vi "Query Outputs.vi"(8 "error in":errorcluster, 11 "PIOD in":refnum<class "PIOD.lvclass">) -> (0 "error out":errorcluster, 3 "PIOD out":refnum<class "PIOD.lvclass">)   [LabVIEW 2018, in "PIOD.lvlib" / "PIOD.lvclass"]
uses:
  PIOD.lvclass
  Custom Controls/File Number.ctl
  PIOD.lvclass/PIOD.ctl
  Accessors/Read/Read Timeout (ms).vi
  <vilib>/ethernetip/ethernetip.llb/EthernetIP SLC500 Read Bit.vi
  <vilib>/ethernetip/ethernetip.lvlib
  PPLs/PLC/Parent/PLC.lvlibp/PLC.lvclass
  C:/AME Test Engineering/LabVIEW/PPLs/PLC/Parent/PLC.lvlibp/PLC.lvclass
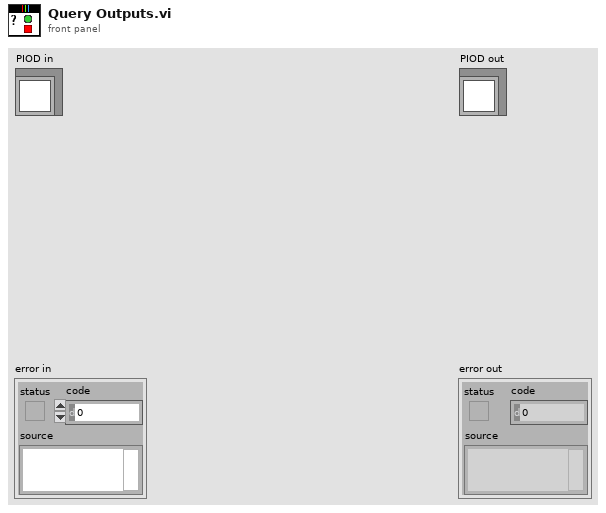
[diagram p1: front panel]
types:
  T1 = typedef "PIOD.lvlib/PIOD.lvclass/File Number.ctl" = enum16{"Output", "Input", "Status", "Output2"}
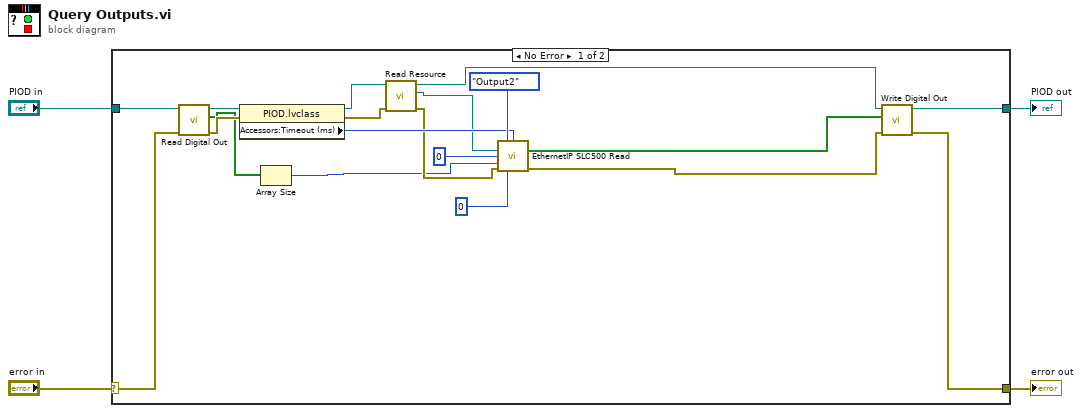
[diagram p0: block diagram]
diagram:
  n1 = case shown="No Error" "error in" {
    selector: "error in" -> [w11 w25]
    tunnel: [w20 w25] -> w3
    tunnel: [w21 w24] -> w1
    tunnel: "PIOD in" -> [w12 w24]
    frame No Error {
      n2 = call "Read Digital Out.vi"("error in"=w11, "PLC in"=w12) -> ("error out"=w9:errorcluster, "Digital Out"=w8:bool[], "PLC out"=w10:refnum<class "PIOD.lvclass">)  [unwired: 7 in]
      n3 = property class="PIOD.lvclass"(reference=w10, error in=w9) -> (reference out=w18:refnum<class "PIOD.lvclass">, error out=w19:errorcluster, "Accessors:Timeout (ms)"=w22:i32)
      n4 = Array Size(array=w8) -> (size(s)=w6:i32)
      n5 = call "Read Resource.vi"("error in (no error)"=w19, "PLC in"=w18) -> ("error out"=w15:errorcluster, "Resource"=w16:refnum<visa-resource-name>, "PLC out"=w17:refnum<class "PIOD.lvclass">)  [unwired: 7 in]
      n6 = call-poly <vilib>:"EthernetIP SLC500 Read.vi"("File Number"=File_Number."Output2", "Timeout (ms)"=w22, "Network Path"=w16, "Element Number"=u16 0, "Number of Bits"=w6, "error in"=w15, "Bit Offset"=u16 0) -> ("Data"=w7:bool[], "error out"=w14:errorcluster)  [unwired: 6 in, 1 out]
      n7 = call "Write Digital Out.vi"("error in (no error)"=w14, "Digital Out"=w7, "PLC in"=w17) -> ("error out"=w20:errorcluster, "PLC out"=w21:refnum<class "PIOD.lvclass">)  [unwired: 7 in]
    }
    frame Error {
    }
  }
  "error out" <- w3
  "PIOD out" <- w1
